vi "GlobalError.vi"() -> ()   [LabVIEW 2017]
uses:
  Globalvalue1.vi
panel:
  in  "stop":bool
  out "Final value":i32
  out "Sum":i32
  in  "Starting value":i32
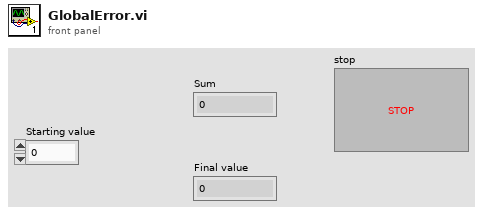
[diagram p1: front panel]
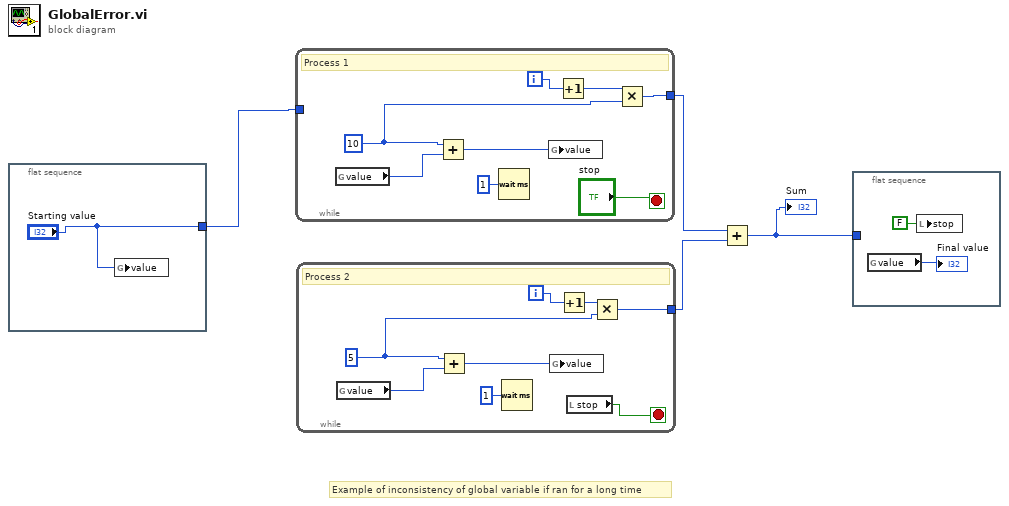
[diagram p0: block diagram]
diagram:
  # "Example of inconsistency of global variable if ran for a long time"
  n1 = flat-sequence {
    tunnel: ["Starting value"] -> w4
    frame #0 {
      n2 = global write "Globalvalue1.vi" "value"("Starting value") -> ()
    }
  }
  n3 = while {
    tunnel: w4 -> [_]
    tunnel: [w8] -> w3
    i -> [w12]
    stop <- "stop" stop-if-true
    w10 = 10
    # "Process 1"
    n4 = global read "Globalvalue1.vi" "value"() -> (w11:i32)
    n5 = Add(x=w10, y=w11) -> (x+y=w9:i32)
    n6 = Wait (ms)(milliseconds to wait=u32 1) -> ()  [unwired: 1 out]
    n7 = global write "Globalvalue1.vi" "value"(w9) -> ()
    n8 = Increment(x=w12) -> (x+1=w13:i32)
    n9 = Multiply(x=w13, y=w10) -> (x*y=w8:i32)
  }
  n10 = while {
    tunnel: [w16] -> w1
    i -> [w20]
    stop <- w14 stop-if-true
    w18 = 5
    # "Process 2"
    n11 = global read "Globalvalue1.vi" "value"() -> (w19:i32)
    n12 = Add(x=w18, y=w19) -> (x+y=w17:i32)
    n13 = Wait (ms)(milliseconds to wait=u32 1) -> ()  [unwired: 1 out]
    n14 = global write "Globalvalue1.vi" "value"(w17) -> ()
    n15 = Increment(x=w20) -> (x+1=w21:i32)
    n16 = local read "stop"() -> (w14:bool)
    n17 = Multiply(x=w21, y=w18) -> (x*y=w16:i32)
  }
  n18 = Add(x=w3, y=w1) -> (x+y=w2:i32)
  "Sum" <- w2
  n19 = flat-sequence {
    tunnel: w2 -> [_]
    frame #0 {
      n20 = global read "Globalvalue1.vi" "value"() -> (→"Final value":i32)
      n21 = local write "stop"(FALSE ("stop")) -> ()
    }
  }
